vi "Teleop.vi"(10 "Match Info":T1={"Autonomous Elapsed Seconds"=0.0, "TeleOp Elapsed Seconds"=0.0, "Disabled Elapsed Seconds"=0.0, "Visited Autonomous"=FALSE, "Visited TeleOp"=FALSE, "Visited Disabled"=FALSE, "Autonomous Settings"={"Autonomous Style"=enum."Independent", "VI Refnum"=refnum}}, 11 "Call Context":T2) -> ()   [LabVIEW 2020]
doc: "This VI is called for each TeleOp packet received from the DS where the robot is not disabled. It is often used to read from the joysticks and update I/O or to update setpoints for timed control loops. It should complete and return within 20 milliseconds or it may miss DS packets."
uses:
  <vilib>/Rock Robotics/WPI/DriverStation/WPI_DriverStationDerivedRobotMode.ctl
  <vilib>/Rock Robotics/WPI/DriverStation/WPI_DriverStationMatch Info.ctl
  <vilib>/Rock Robotics/WPI/Utilities/WPI_GetSetVariantRefNum.vi
  Robot Global Data.vi
  <vilib>/Rock Robotics/Network Tables/NT Read Boolean.vi
  <vilib>/Rock Robotics/Network Tables/NT Read Number.vi
panel:
  out "Sample Slider 0":dbl(slide) scale=0.0..5.0
  out "Sample Boolean 1":bool
  out "Sample Boolean 0":bool
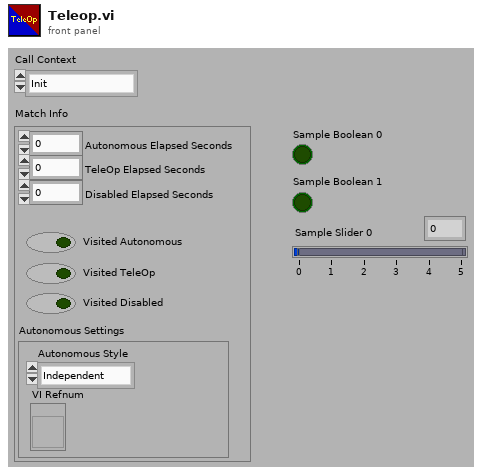
[diagram p1: front panel]
types:
  T1 = typedef "WPI_DriverStationMatch Info.ctl" = cluster{"Autonomous Elapsed Seconds":dbl, "TeleOp Elapsed Seconds":dbl, "Disabled Elapsed Seconds":dbl, "Visited Autonomous":bool, "Visited TeleOp":bool, "Visited Disabled":bool, "Autonomous Settings":cluster{"Autonomous Style":enum16{"Iterative", "Independent"}, "VI Refnum":refnum<vi>}}
  T2 = typedef "WPI_DriverStationDerivedRobotMode.ctl" = enum16{"Init", "Execute", "Stop"}
  T3 = typedef "WPI_JoystickDevRef.ctl" = cluster{"Device":T4}
  T4 = typedef "WPI_JoystickDeviceEnum.ctl" = enum16{"USB 0", "USB 1", "USB 2", "USB 3", "USB 4", "USB 5"}
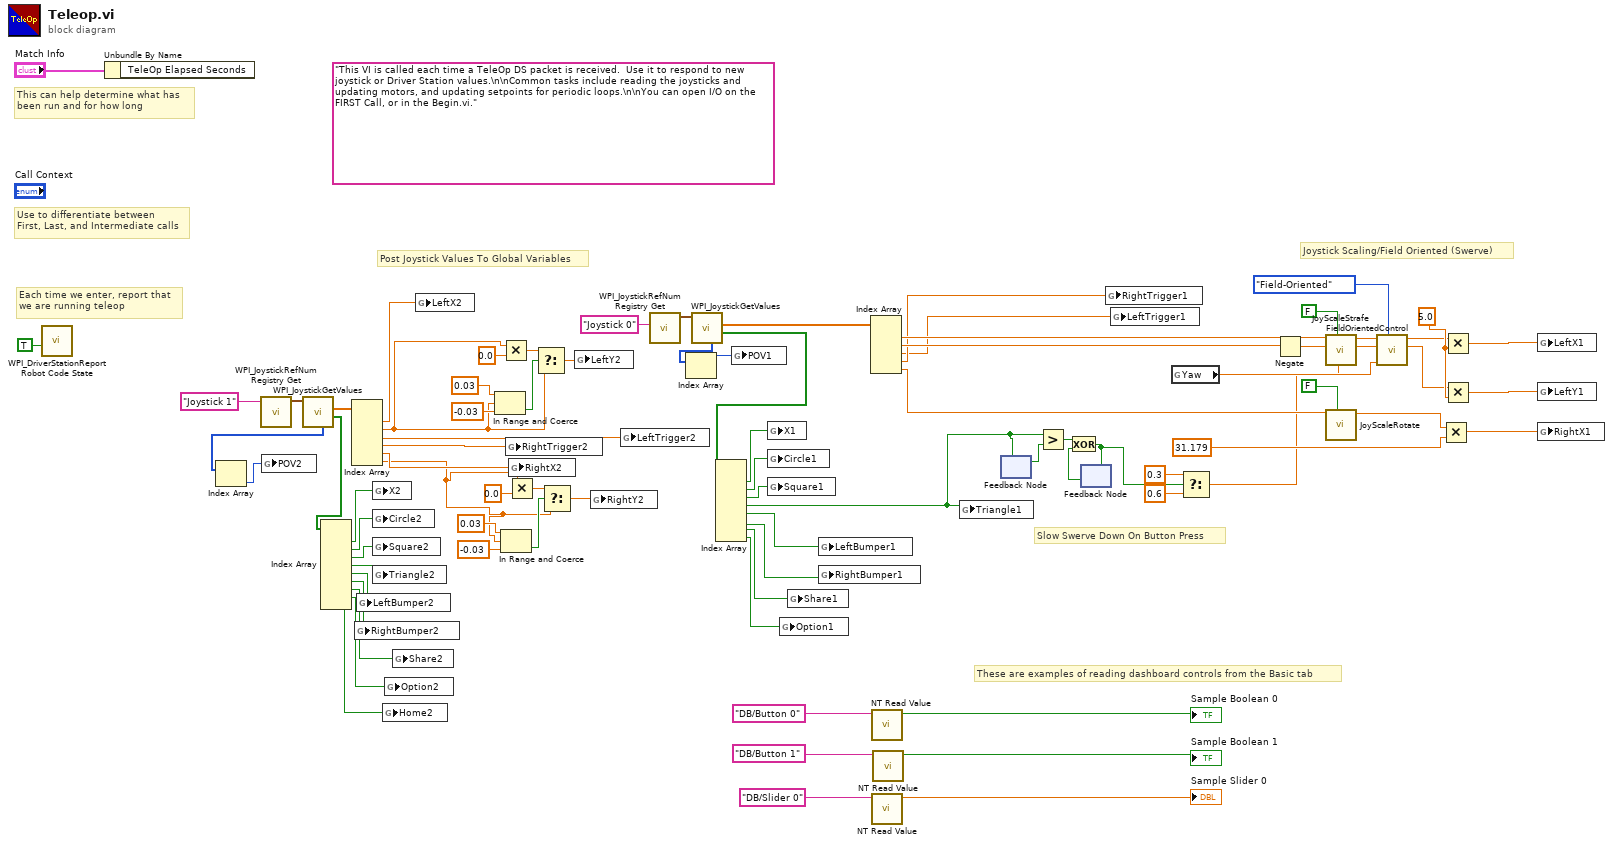
[diagram p0: block diagram]
diagram:
  w61 = 5.0 ("y")
  (unwired) "This VI is called each time a TeleOp DS packet is received.  Use it to respond to new joystick or Driver Station values.\n\nCommon tasks include reading the joysticks and updating motors, and updating setpoints for periodic loops.\n\nYou can open I/O on the FIRST Call, or in the Begin.vi."
  # "Slow Swerve Down On Button Press"
  # "Joystick Scaling/Field Oriented (Swerve)"
  # "Post Joystick Values To Global Variables"
  # "These are examples of reading dashboard controls from the Basic tab"
  # "Each time we enter, report that\nwe are running teleop"
  # "Use to differentiate between\nFirst, Last, and Intermediate calls"
  # "This can help determine what has\nbeen run and for how long"
  n1 = call <vilib>:"WPI_DriverStationReport Robot Code State.vi"("TeleOp"=TRUE ("Autonomous")) -> ()  [unwired: 10 in, 1 out]
  n2 = Unbundle By Name("Match Info") -> ()  [unwired: 1 out]
  n3 = call <vilib>:"WPI_JoystickRefNum Registry Get.vi"("refnum name"="Joystick 1") -> ("JoystickDevRef"=w65:T3)  [unwired: 1 in, 9 out]
  n4 = call <vilib>:"WPI_JoystickGetValues.vi"("JoystickDevRef"=w65) -> ("Buttons"=w34:bool[], "Axes"=w63:dbl[], "POVs"=w33:i16[])  [unwired: 6 in, 2 out]
  n5 = Index Array(array=w33) -> (element=w32:i16)  [unwired: 1 in]
  n6 = global write "Robot Global Data.vi" "POV2"(w32) -> ()
  n7 = Index Array(array=w34) -> (element #1=w35:bool, element #2=w36:bool, element #3=w37:bool, element #4=w38:bool, element #5=w39:bool, element #6=w40:bool, element #7=w41:bool, element #8=w42:bool, element #9=w31:bool)  [unwired: 9 in]
  n8 = Index Array(array=w63) -> (element #1=w44:dbl, element #2=w9:dbl, element #3=w45:dbl, element #4=w46:dbl, element #5=w43:dbl, element #6=w1:dbl)  [unwired: 6 in]
  n9 = global write "Robot Global Data.vi" "RightBumper2"(w40) -> ()
  n10 = global write "Robot Global Data.vi" "LeftBumper2"(w39) -> ()
  n11 = global write "Robot Global Data.vi" "X2"(w35) -> ()
  n12 = global write "Robot Global Data.vi" "Circle2"(w36) -> ()
  n13 = global write "Robot Global Data.vi" "Square2"(w37) -> ()
  n14 = global write "Robot Global Data.vi" "Triangle2"(w38) -> ()
  n15 = global write "Robot Global Data.vi" "Home2"(w31) -> ()
  n16 = global write "Robot Global Data.vi" "Option2"(w42) -> ()
  n17 = global write "Robot Global Data.vi" "Share2"(w41) -> ()
  n18 = global write "Robot Global Data.vi" "LeftX2"(w44) -> ()
  n19 = In Range and Coerce(upper limit=0.03, x=w9, lower limit=-0.03) -> (In Range?=w10:bool)  [unwired: 1 out]
  n20 = Multiply(x=w9, y=0.0) -> (x*y=w11:dbl)
  n21 = In Range and Coerce(upper limit=0.03, x=w1, lower limit=-0.03) -> (In Range?=w3:bool)  [unwired: 1 out]
  n22 = global write "Robot Global Data.vi" "RightTrigger2"(w46) -> ()
  n23 = Multiply(x=w1, y=0.0) -> (x*y=w4:dbl)
  n24 = global write "Robot Global Data.vi" "RightX2"(w43) -> ()
  n25 = Select(t=w11, s=w10, f=w9) -> (s? t:f=w8:dbl)
  n26 = Select(t=w4, s=w3, f=w1) -> (s? t:f=w2:dbl)
  n27 = global write "Robot Global Data.vi" "LeftY2"(w8) -> ()
  n28 = global write "Robot Global Data.vi" "RightY2"(w2) -> ()
  n29 = global write "Robot Global Data.vi" "LeftTrigger2"(w45) -> ()
  n30 = call <vilib>:"WPI_JoystickRefNum Registry Get.vi"("refnum name"="Joystick 0") -> ("JoystickDevRef"=w80:T3)  [unwired: 1 in, 9 out]
  n31 = call <vilib>:"WPI_JoystickGetValues.vi"("JoystickDevRef"=w80) -> ("Buttons"=w57:bool[], "Axes"=w78:dbl[], "POVs"=w48:i16[])  [unwired: 6 in, 2 out]
  n32 = Index Array(array=w48) -> (element=w47:i16)  [unwired: 1 in]
  n33 = Index Array(array=w57) -> (element #1=w58:bool, element #2=w56:bool, element #3=w55:bool, element #4=w19:bool, element #5=w54:bool, element #6=w51:bool, element #7=w50:bool, element #8=w49:bool)  [unwired: 8 in]
  n34 = global write "Robot Global Data.vi" "POV1"(w47) -> ()
  n35 = global write "Robot Global Data.vi" "X1"(w58) -> ()
  n36 = global write "Robot Global Data.vi" "Circle1"(w56) -> ()
  n37 = global write "Robot Global Data.vi" "Square1"(w55) -> ()
  n38 = global write "Robot Global Data.vi" "Option1"(w49) -> ()
  n39 = global write "Robot Global Data.vi" "Share1"(w50) -> ()
  n40 = global write "Robot Global Data.vi" "LeftBumper1"(w54) -> ()
  n41 = global write "Robot Global Data.vi" "RightBumper1"(w51) -> ()
  n42 = Index Array(array=w78) -> (element #1=w71:dbl, element #2=w70:dbl, element #3=w52:dbl, element #4=w53:dbl, element #5=w67:dbl)  [unwired: 5 in]
  n43 = call-poly <vilib>:"NT Read Value.vi"("name"="DB/Button 0" ("refnum name")) -> ("value"=→"Sample Boolean 0":bool)  [unwired: 8 in, 2 out]
  n44 = call-poly <vilib>:"NT Read Value.vi"("name"="DB/Slider 0" ("refnum name")) -> ("value"=→"Sample Slider 0":dbl)  [unwired: 8 in, 2 out]
  n45 = call-poly <vilib>:"NT Read Value.vi"("name"="DB/Button 1" ("refnum name")) -> ("value"=→"Sample Boolean 1":bool)  [unwired: 8 in, 2 out]
  n46 = global write "Robot Global Data.vi" "Triangle1"(w19) -> ()
  n47 = feedback #1() -> (w20:bool)  [unwired: 1 in]
  n48 = feedback-in #1(w19) -> ()
  n49 = Greater?(x=w19, y=w20) -> (0:w22:bool)
  n50 = feedback #2() -> (w21:bool)  [unwired: 1 in]
  n51 = Exclusive Or(1:w21, 2:w22) -> (0:w18:bool)
  n52 = feedback-in #2(w18) -> ()
  n53 = global write "Robot Global Data.vi" "RightTrigger1"(w53) -> ()
  n54 = global write "Robot Global Data.vi" "LeftTrigger1"(w52) -> ()
  n55 = global read "Robot Global Data.vi" "Yaw"() -> (w60:dbl)
  n56 = Select(t=0.3, s=w18, f=0.6) -> (s? t:f=w17:dbl)
  n57 = Negate(x=w70) -> (-x=w23:dbl)
  n58 = call "JoyScaleStrafe.vi"("Strafe Maximum"=w17, "Auto Control"=FALSE, "Raw Joystick Y"=w23, "Raw Joystick X"=w71) -> ("Scaled Joystick Y"=w27:dbl, "Scaled Joystick X"=w26:dbl)  [unwired: 5 in, 1 out]
  n59 = call "JoyScaleRotate.vi"("Auto Control"=FALSE, "Raw Joystick Rotation"=w67) -> ("Scaled Joystick Rotation"=w30:dbl)  [unwired: 8 in, 1 out]
  n60 = call "FieldOrientedControl.vi"("Orientation Mode"=enum16{"Robot-Oriented", "Field-Oriented"}."Field-Oriented", "Robot_H (deg)"=w60, "Joystick Y"=w27, "Joystick X"=w26) -> ("Joystick Y'"=w29:dbl, "Joystick X'"=w28:dbl)  [unwired: 6 in]
  n61 = Multiply(x=w30, y=31.179 ("x")) -> (x*y=w66:dbl)
  n62 = Multiply(x=w28, y=w61) -> (x*y=w68:dbl)
  n63 = Multiply(x=w29, y=w61) -> (x*y=w69:dbl)
  n64 = global write "Robot Global Data.vi" "LeftX1"(w68) -> ()
  n65 = global write "Robot Global Data.vi" "LeftY1"(w69) -> ()
  n66 = global write "Robot Global Data.vi" "RightX1"(w66) -> ()
